vi "Post-Dig.vi"(6 "Call and Forget?":bool, 8 "Error In":errorcluster, 10 "Grave In":refnum<vi>, 11 "VI In":refnum<vi>) -> (0 "Error Out":errorcluster, 2 "Grave Out":refnum<vi>, 3 "VI Out":refnum<vi>)   [LabVIEW 2018, in "Tests.lvlib" / "Toolkit.lvlib" / "Integration.lvlib"]
uses:
  Integration.lvlib
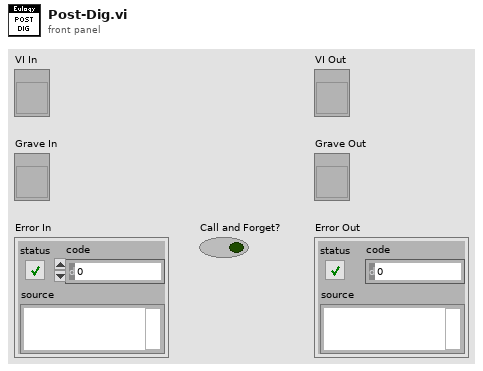
[diagram p1: front panel]
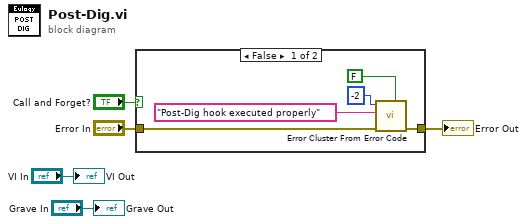
[diagram p0: block diagram]
diagram:
  n1 = case shown="False" "Call and Forget?" {
    tunnel: [w10 w11] -> w4
    tunnel: "Error In" -> [w9 w11]
    frame False {
      n2 = call <vilib>:"Error Cluster From Error Code.vi"("is warning? (False)"=FALSE, "error in (no error)"=w9, "error message (\"\")"="Post-Dig hook executed properly" ("error message (\"\")"), "error code (0)"=-2) -> ("error out"=w10:errorcluster)  [unwired: 5 in]
    }
    frame True {
    }
  }
  "Error Out" <- w4
  "VI Out" <- "VI In"
  "Grave Out" <- "Grave In"
